vi "Configure Standard Waveform Advanced (Square).vi"(8 "error in (no error)":errorcluster, 9 "Duty Cycle (50 Percent)":dbl=50.0, 10 "Channel (1: 1)":i32(ring)=1 items=["1"=1, "2"=2], 11 "VISA resource name":refnum<visa-resource-name>) -> (0 "error out":errorcluster, 3 "VISA resource name out":refnum<visa-resource-name>)   [LabVIEW 2026, in "Agilent 3352X Series.lvlib"]
doc: "Sets duty cycle parameters for square waveform.\nDuty cycle represents the amount of time per cycle that the square wave is at a high level (assuming that the waveform polarity is not inverted). \n\n<b>Note</b>:\n(1) This VI is only used to work with Configure Standard Waveform.VI when waveform function set to be Square\n(2) The duty cycle setting is remembered when you change from square wave to another function. When you return to the square wave function, the previous duty cycle is used. \n(3) If you select a square waveform as the modulating waveform for AM, FM, PM, or PWM, the duty cycle setting does not apply. The waveform generator always uses a square waveform with a 50% duty cycle."
uses:
  Agilent 3352X Series.lvlib
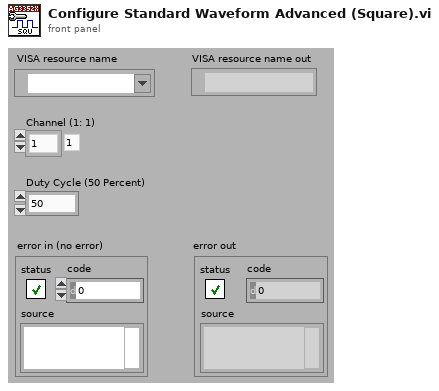
[diagram p1: front panel]
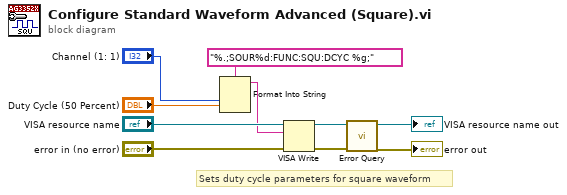
[diagram p0: block diagram]
diagram:
  # "Sets duty cycle parameters for square waveform"
  n1 = Format Into String(format string="%.;SOUR%d:FUNC:SQU:DCYC %g;", "Channel (1: 1)", "Duty Cycle (50 Percent)") -> (resulting string=w1:string)  [unwired: 2 in, 1 out]
  n2 = VISA Write(VISA resource name="VISA resource name", write buffer=w1, error in (no error)="error in (no error)") -> (VISA resource name out=w5:refnum<visa-resource-name>, error out=w4:errorcluster)  [unwired: 1 out]
  n3 = call "Error Query.vi"("error in (no error)"=w4, "VISA resource name"=w5) -> ("error out"=→"error out":errorcluster, "VISA resource name out"=→"VISA resource name out":refnum<visa-resource-name>)  [unwired: 8 out]
